vi "GV PreframegateRescanGalvo.vi"() -> ()   [LabVIEW 2017]
panel:
  out "PreframegateRescanGalvo":bool
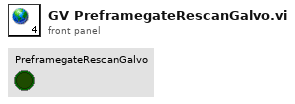
[diagram p1: front panel]
diagram:
